vi "Version.vi"(8 "error in (no error)":errorcluster, 11 "Builder in":refnum<class "Builder.lvclass">) -> (0 "error out":errorcluster, 2 "Version":T1, 3 "Builder out":refnum<class "Builder.lvclass">)   [LabVIEW 2020, in "Builder Tools.lvlib" / "Builder.lvclass"]
uses:
  Builder.lvclass
  Builder.lvclass/Builder.ctl
  <vilib>/AppBuilder/AB_API_Simple/NI_App_Builder_API.lvlib
  <vilib>/AppBuilder/AB_API_Simple/Get Build Specification Version (path).vi
  Builder Core/Version.ctl
  Builder Core/Builder Core.lvlib
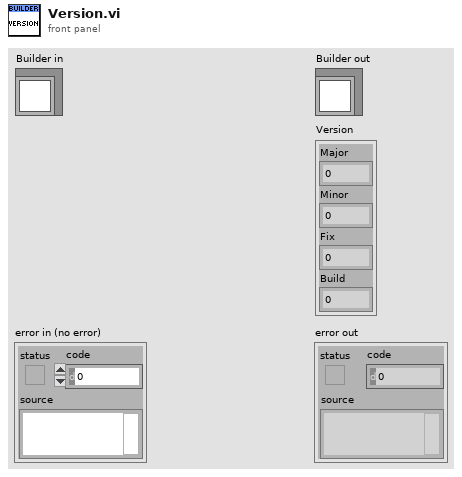
[diagram p1: front panel]
types:
  T1 = typedef "Builder Core.lvlib/Version.ctl" = cluster{"Major":u16, "Minor":u16, "Fix":u16, "Build":u16}
  T2 = typedef "Builder Tools.lvlib/Builder.lvclass/Build Step.ctl" = cluster{"Info":T3, "Build":refnum<class "Build.lvclass">}
  T3 = typedef "Builder Tools.lvlib/Build Info.ctl" = cluster{"Project Path":path, "Target":string, "Build Spec":string}
  T4 = typedef "NI_App_Builder_API.lvlib/Build Specification Version.ctl" = cluster{"Major":u16, "Minor":u16, "Fix":u16, "Build":u16}
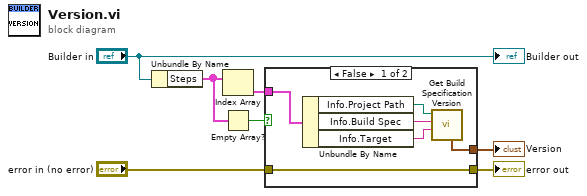
[diagram p0: block diagram]
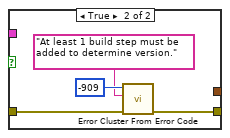
[diagram p2: hidden frame]
diagram:
  n1 = Unbundle By Name("Builder in") -> ("Steps"=w6:T2[])
  n2 = Index Array(array=w6) -> (element=w5:T2)  [unwired: 1 in]
  n3 = Empty Array?(array=w6) -> (empty?=w4:bool)
  n4 = case shown="False" w4 {
    tunnel: w5 -> [w12 _]
    tunnel: "error in (no error)" -> [w13 w17]
    tunnel: [w13 w16] -> w2
    tunnel: [w8 _] -> w1
    frame False {
      n5 = Unbundle By Name(w12) -> ("Info.Project Path"=w11:path, "Info.Build Spec"=w10:string, "Info.Target"=w9:string)
      n6 = call-poly <vilib>:"Get Build Specification Version.vi"("Name of target (My Computer)"=w9, "Name of build specification"=w10, "Path to project"=w11) -> ("Build Specification Version"=w8:T4)  [unwired: 7 in, 1 out]
    }
    frame True {
      n7 = call <vilib>:"Error Cluster From Error Code.vi"("error in (no error)"=w17, "error message (\"\")"="At least 1 build step must be added to determine version.", "error code (0)"=-909) -> ("error out"=w16:errorcluster)  [unwired: 6 in]
    }
  }
  "error out" <- w2
  "Version" <- w1
  "Builder out" <- "Builder in"
